vi "FFT on FPGA (BUGGED!).vi"   [LabVIEW 2014]
uses:
  <vilib>/Platform/TimedLoop/XDataNode/timing_clust.ctl
  <vilib>/Platform/TimedLoop/XDataNode/nitl_modes.ctl
  <vilib>/Platform/TimedLoop/XDataNode/wakeup.ctl
  <vilib>/rvi/Analysis/measure/FFT/simModelSupport/niFPGA FFT Streaming Sim Properties.ctl
  <vilib>/rvi/Analysis/measure/FFT/simModelSupport/niFPGA FFT Sim Stream Group Properties.ctl
  <vilib>/rvi/Analysis/measure/FFT/simModelSupport/niFPGA FFT Sim Types.ctl
  <vilib>/rvi/Analysis/measure/FFT/simModelSupport/niFpgaFFTSimArithmeticProperties.ctl
  <vilib>/rvi/Analysis/measure/FFT/simModelSupport/niFpgaFFTSimDfxp.ctl
  <vilib>/fxp/LVFixedPointQuantizationPolicyTypeDef.ctl
  <vilib>/rvi/Analysis/measure/FFT/XNode/niFpgaFFTButterflyDelays.ctl
  <vilib>/rvi/Emulation/niFpgaSctlEmulationGetInTimedLoop.vi
  <vilib>/rvi/Emulation/niFpgaEmulationReportErrorSimple.vi
  <vilib>/rvi/Emulation/niFpgaGetClockAttributes.vi
  <vilib>/rvi/Emulation/niFpgaCriticalErrorInLSC.vi
  <vilib>/rvi/Emulation/niFpgaEmulationIsFPGAContextNoSignature.vi
  <vilib>/rvi/errors/niFpgaSetErrorForExecOnDevCompSimple.vi
  <vilib>/rvi/eio/common/nirviEmuReportErrorAndStop.vi
  <vilib>/rvi/DataTransferAndStorage/Container/Common/niFpgaContainerGetUniqueNameForEmu.vi
  <vilib>/rvi/FIFO/Fifo_Resource/nirvififoEmulationSetSize.vi
  <vilib>/rvi/FIFO/Fifo_Resource/nirviFifoEmulationQueueMgr.vi
  <instcachedir>/0/nirviFifoEmulationQueueMgr_E5CAEC123FF24DC58D834DCA3CDAA9B5.lvgen/nirviFifoEmulationQueueMgr_E5CAEC123FF24DC58D834DCA3CDAA9B5_012.vi
  <vilib>/rvi/FIFO/Fifo_Resource/nirvififoEmulationCreateLock.vi
  <vilib>/rvi/Emulation/niFpgaProcessEmulError.vi
  <vilib>/rvi/FIFO/Fifo_Resource/nirvififoEmulationObtainLock.vi
  <vilib>/rvi/FIFO/Fifo_Resource/nirvififoEmulationReleaseLock.vi
  <vilib>/rvi/occurrence/nirviWaitOnOccurrenceBase.vi
  <vilib>/rvi/errors/nirviReportUnexpectedCaseInternalError.vi
  <vilib>/rvi/errors/nirviReportUnexpectedCaseInternalError (U32).vi
  <vilib>/rvi/Memory/Memory_Emulation/niFpgaMemoryEmulationCacheClearOnFirstRun.vi
  <vilib>/rvi/Memory/Memory_Emulation/nirvimemoryEmulationManagerCache_MakeExclusive.vi
  <vilib>/rvi/Memory/Memory_Emulation/niFpgaMemoryEmulationValidateCache.vi
  <vilib>/rvi/Memory/Memory_Emulation/nirvimemoryEmulationManagerCache_InsertValue.vi
  <vilib>/Utility/error.llb/Clear Errors.vi
  <vilib>/rvi/Memory/Memory_Emulation/nirvimemoryEmulationManagerCache_ReleaseExclusive.vi
  <vilib>/rvi/Memory/Memory_Emulation/nirvimemoryEmulationManagerCache_GetValue.vi
  <vilib>/rvi/Memory/Memory_Emulation/nirvimemoryEmulationManagerCache_SetValue.vi
  <instcachedir>/0/nirviFifoEmulationQueueMgr_E5CAEC123FF24DC58D834DCA3CDAA9B5.lvgen/nirviFifoEmulationQueueMgr_E5CAEC123FF24DC58D834DCA3CDAA9B5_010.vi
  <vilib>/rvi/eio/common/nirviEmuTemplateMethod_errors.vi
  <vilib>/rvi/FIFO/Fifo_Resource/nirvififoEmulationDetermineInputValidOut.vi
  <vilib>/rvi/Memory/Memory_Emulation/nirvimemoryFastEmulation.vi
  <vilib>/rvi/Memory/Memory_Emulation/nirvimemoryEmulation.vi
  <vilib>/rvi/interface/RandomDataEmulation/niFpgaRandomDataHandleErrors.vi
  <vilib>/rvi/Analysis/measure/FFT/simModelSupport/niFpgaFFTSimModelStreamingCore.vi
  <vilib>/Platform/TimedLoop/XDataNode/XDataNode.xnode
  <vilib>/rvi/DataTransferAndStorage/Container/XNode/niFpgaContainer.xnode
  <vilib>/rvi/FIFO/Fifo_Resource/nirvififoEmulationRead.vi
  <vilib>/rvi/DataTransferAndStorage/Register/Emulation/niFpgaRegisterEmulation.vi
  <vilib>/eio/EIOMethodNode/EIOMethodNode.xnode
  <vilib>/rvi/FIFO/Fifo_Resource/nirvififoEmulationWrite.vi
  <vilib>/rvi/interface/RandomDataEmulation/nirviRandomDataFpgaReadWriteTemplate.vi
  <vilib>/rvi/Analysis/measure/FFT/XNode/niFpgaFFT.xnode
  <vilib>/Platform/TimedLoop/XDataNode/XDNodeRunTimeDep.lvlib
types:
  T1 = typedef "XDNodeRunTimeDep.lvlib/timing_clust.ctl" = cluster{"Expected End [f-1]":u64, "Actual End [f-1]":u64, "Finished Late? [f-1]":bool, "Expected End [i-1]":u64, "Actual End [i-1]":u64, "Finished Late? [i-1]":bool, "Expected Start [i]":u64, "Actual Start [i]":u64, "Expected Start [f]":u64, "Actual Start [f]":u64, "Source Name":string, "Structure Name":string, "Period":i64, "Deadline":i64, "Offset":i64, "Start":i64, "Priority":i32, "Timeout":i32, "Mode":T2, "Wakeup Reason":T3, "Error":errorcluster, "Source Type":string, "Secondary Source Type":string, "Global End Time":u64, "Global Start Time":u64, "Frame Duration":u64, "Iteration Duration":u64, "Assigned CPU":i32, "I/O Scan Engine Mode":u32}
  T2 = typedef "XDNodeRunTimeDep.lvlib/nitl_modes.ctl" = enum32{"No Change", "Process missed periods, maintain original phase", "Discard missed periods, maintain original phase", "Process missed periods, ignore original phase", "Discard missed periods, ignore original phase"}
  T3 = typedef "XDNodeRunTimeDep.lvlib/wakeup.ctl" = enum32{"Normal", "Aborted", "Asynchronous wakeup", "Timing source error", "Timed loop error", "Timeout"}
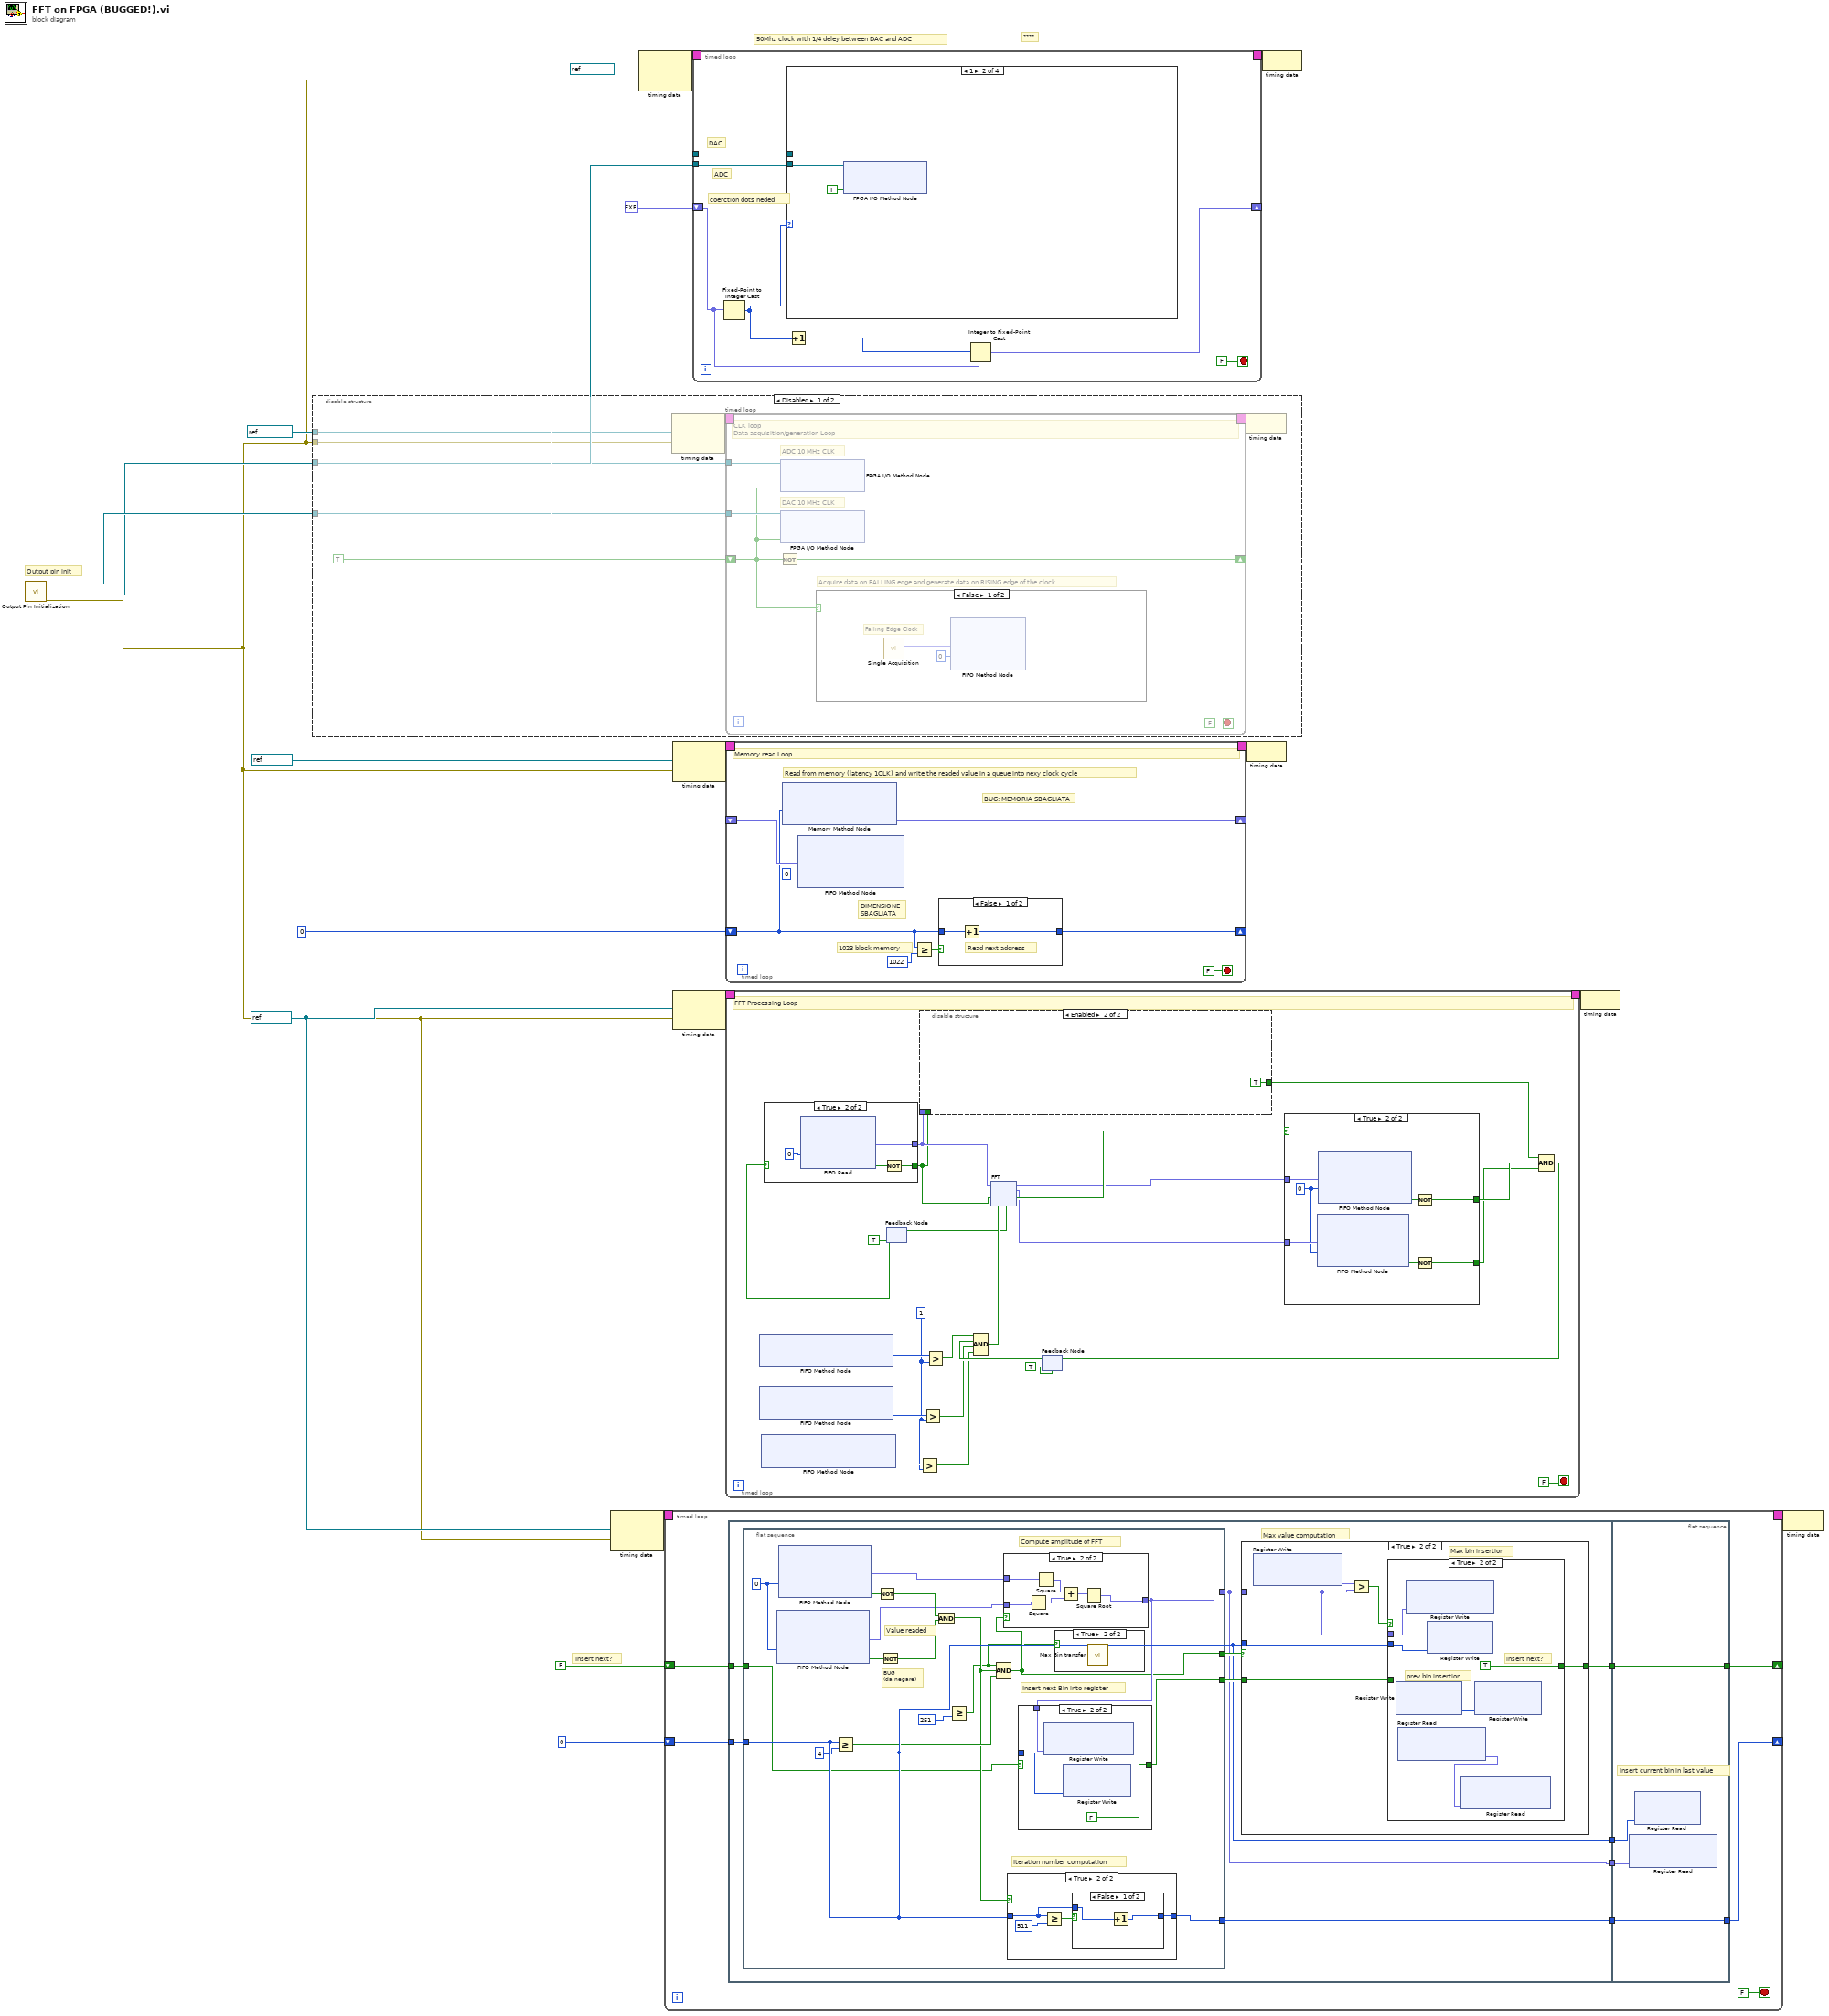
[diagram p0: block diagram]
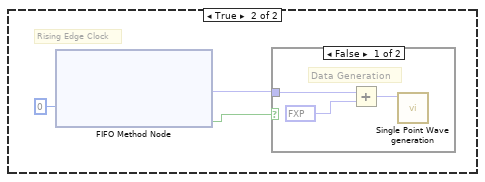
[diagram p2: hidden frame]
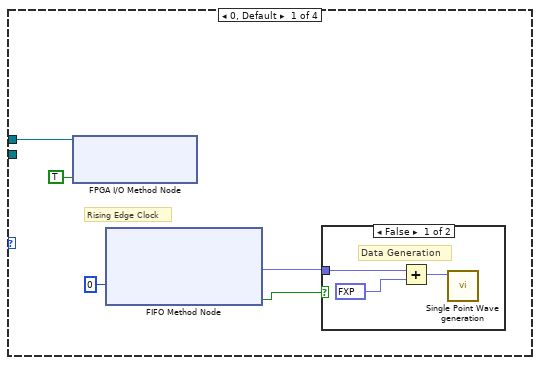
[diagram p5: hidden frame]
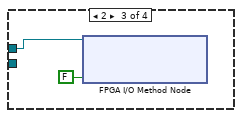
[diagram p7: hidden frame]
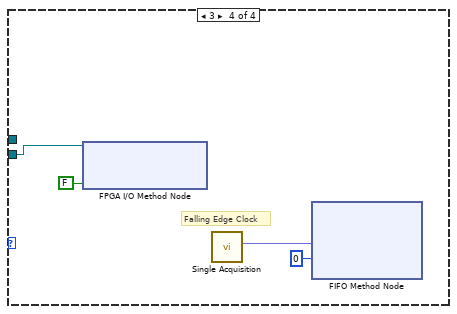
[diagram p8: hidden frame]
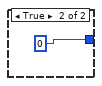
[diagram p12: hidden frame]
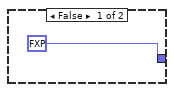
[diagram p13: hidden frame]
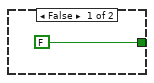
[diagram p15: hidden frame]
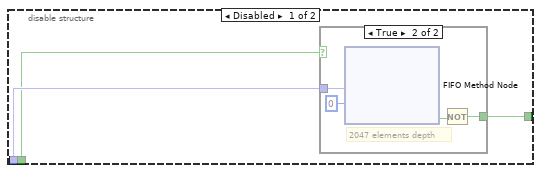
[diagram p16: hidden frame]
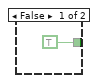
[diagram p17: hidden frame]
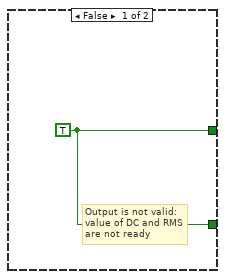
[diagram p18: hidden frame]
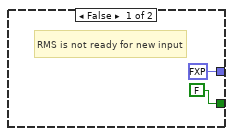
[diagram p19: hidden frame]
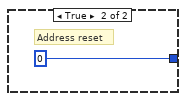
[diagram p20: hidden frame]
diagram:
  w10 = refnum<k21> "50MHz" ("Source Name")
  # "????"
  # "50Mhz clock with 1/4 deley between DAC and ADC"
  # "Insert next?"
  # "Output pin init"
  n1 = call "Output Pin Initialization.vi"() -> ("error out"=w1:errorcluster, "I/O Out Clock DAC (pin16)"=w2:refnum<k21>, "I/O Out Clock ADC (pin17)"=w3:refnum<k21>)  [unwired: 8 in]
  n2 = disable-structure shown="Disabled" {
    disable-tunnel: w1 -> [w23 _]
    disable-tunnel: refnum<k21> "100MHz" ("Source Name") -> [w22 _]
    disable-tunnel: w3 -> [w21 _]
    disable-tunnel: w2 -> [w20 _]
    frame Disabled {
      n3 = node-c288(w22, w23) -> (w26:T1)
      n4 = timed-loop {
        timing: w26 -> [_]
        timing-out: [_] -> w25
        shift-right: [w29] -> _
        shift-left: TRUE -> [w27]
        tunnel: w20 -> [w31]
        tunnel: w21 -> [w28]
        stop <- FALSE stop-if-true
        # "DAC 10 MHz CLK"
        # "Acquire data on FALLING edge and generate data on RISING edge of the clock"
        # "ADC 10 MHz CLK"
        # "CLK loop\nData acquisition/generation Loop"
        n5 = Not(x=w27) -> (.not. x?=w29:bool)
        n6 = xnode "FPGA I/O Method Node"("FPGA I/O In"=w31, "Data"=w27) -> ()  [unwired: 1 out]
        n7 = xnode "FPGA I/O Method Node"("FPGA I/O In"=w28, "Data"=w27) -> ()  [unwired: 1 out]
        n8 = case shown="False" w27 {
          frame False {
            # "Falling Edge Clock"
            n9 = call "Single Acquisition.vi"() -> ("Out"=w32:fxp<+/-,12,12>)  [unwired: 10 in, 1 out]
            n10 = xnode ("FIFO Method Node")("Element"=w32, "Timeout"=0) -> ()  [unwired: 1 in, 2 out]
          }
          frame True {
            # "Rising Edge Clock"
            n11 = xnode ("FIFO Method Node")("Timeout"=0) -> ("Element"=w34:fxp<+/-,12,12>, "Timed Out?"=w35:bool)  [unwired: 1 in, 1 out]
            n12 = case shown="False" w35 {
              tunnel: w34 -> [w39 _]
              frame False {
                # "Data Generation"
                n13 = Add(x=w39, y=fxp<+,12,12> 2048.0) -> (x+y=w37:fxp<+/-,14,14>)
                n14 = call "Single Point Wave generation.vi"("Data To Write"=w37) -> ()  [unwired: 10 in, 1 out]
              }
              frame True {
                # "FPGA memory slow"
              }
            }
          }
        }
      }
      n15 = node-c288(w25) -> ()
    }
    frame Enabled {
    }
  }
  n16 = node-c288(w10, w1) -> (w13:T1)
  n17 = node-c288(refnum<k21> "200MHz" ("Source Name"), w1) -> (w8:T1)
  n18 = timed-loop {
    timing: w13 -> [_]
    timing-out: [_] -> w12
    shift-right: [w54] -> _
    shift-left: 0 ("Timeout") -> [w51]
    shift-right: [w53] -> _
    shift-left: FALSE -> [w52]
    stop <- FALSE stop-if-true
    n19 = flat-sequence {
      tunnel: [w61] -> w49
      tunnel: [w60] -> w48
      tunnel: [w56] -> w47
      tunnel: [w57] -> w50
      tunnel: w52 -> [w59]
      tunnel: w51 -> [w57]
      tunnel: [w115] -> w53
      tunnel: [w116] -> w54
      tunnel: w49 -> [w116]
      tunnel: w48 -> [w115]
      tunnel: w47 -> [w114]
      tunnel: w50 -> [w113]
      frame #0 {
        # "Max value computation"
        n20 = flat-sequence {
          tunnel: [w65] -> w62
          tunnel: [w71] -> w61
          tunnel: w59 -> [w63]
          tunnel: [w68] -> w58
          tunnel: [w67] -> w56
          tunnel: w57 -> [w66]
          frame #0 {
            w80 = 0 ("Timeout")
            # "BUG\n(da negare)"
            # "Iteration number computation"
            # "Insert next Bin into register"
            # "Compute amplitude of FFT"
            # "Value readed"
            n21 = xnode ("FIFO Method Node")("Timeout"=w80) -> ("Element"=w69:fxp<+/-,22,22>, "Timed Out?"=w78:bool)  [unwired: 1 in, 1 out]
            n22 = xnode ("FIFO Method Node")("Timeout"=w80) -> ("Element"=w75:fxp<+/-,22,22>, "Timed Out?"=w79:bool)  [unwired: 1 in, 1 out]
            n23 = Greater Or Equal?(x=w66, y=4) -> (x >= y?=w73:bool)
            n24 = Not(x=w79) -> (.not. x?=w77:bool)
            n25 = Not(x=w78) -> (.not. x?=w76:bool)
            n26 = And(x=w77, y=w76) -> (x .and. y?=w72:bool)
            n27 = Greater Or Equal?(x=w66, y=251) -> (x >= y?=w64:bool)
            n28 = Compound Arithmetic op=AND(w64, w72, w73) -> (w65:bool)
            n29 = case shown="True" w65 {
              tunnel: w75 -> [_ w99]
              tunnel: w69 -> [_ w98]
              tunnel: [fxp<+,46,22> 0.0 w94] -> w67
              frame False {
              }
              frame True {
                n30 = Square(x=w98) -> (x^2=w96:fxp<+,43,43>)
                n31 = Square(x=w99) -> (x^2=w97:fxp<+,43,43>)
                n32 = Add(x=w97, y=w96) -> (x+y=w95:fxp<+,44,44>)
                n33 = Square Root(x=w95) -> (sqrt(x)=w94:fxp<+,46,22>)
              }
            }
            n34 = case shown="True" w72 {
              tunnel: w66 -> [w85 w87]
              tunnel: [w85 w86] -> w71
              frame False {
              }
              frame True {
                n35 = Greater Or Equal?(x=w87, y=511) -> (x >= y?=w89:bool)
                n36 = case shown="False" w89 {
                  tunnel: w87 -> [w90 _]
                  tunnel: [w91 0 ("Timeout")] -> w86
                  frame False {
                    n37 = Increment(x=w90) -> (x+1=w91:i32)
                  }
                  frame True {
                  }
                }
              }
            }
            n38 = case shown="True" w63 {
              selector: w63 -> [w81 _]
              tunnel: [w81 FALSE] -> w68
              tunnel: w67 -> [_ w83]
              tunnel: w66 -> [_ w84]
              frame False {
              }
              frame True {
                n39 = xnode "Register Write"("Data"=w83) -> ()  [unwired: 1 in, 1 out]
                n40 = xnode "Register Write"("Data"=w84) -> ()  [unwired: 1 in, 1 out]
              }
            }
            n41 = case shown="True" w64 {
              frame False {
              }
              frame True {
                n42 = call "Max Bin transfer.vi"() -> ()  [unwired: 11 in, 1 out]
              }
            }
          }
        }
        n43 = case shown="True" w62 {
          tunnel: w56 -> [_ w104]
          tunnel: w57 -> [_ w103]
          tunnel: [w100 w102] -> w60
          tunnel: w58 -> [w100 w101]
          frame False {
          }
          frame True {
            # "Max bin insertion"
            n44 = xnode "Register Write"() -> ("Data"=w106:fxp<+,46,22>)  [unwired: 1 in, 1 out]
            n45 = Greater?(x=w106, y=w104) -> (0:w105:bool)
            n46 = case shown="True" w105 {
              tunnel: w104 -> [_ w112]
              tunnel: w103 -> [_ w111]
              tunnel: [FALSE TRUE] -> w102
              tunnel: w101 -> [_ _]
              frame False {
              }
              frame True {
                # "insert next?"
                # "prev bin insertion"
                n47 = xnode "Register Write"() -> ("Data"=w109:i32)  [unwired: 1 in, 1 out]
                n48 = xnode "Register Read"() -> ("Data"=w108:fxp<+,46,22>)  [unwired: 1 in, 1 out]
                n49 = xnode "Register Write"("Data"=w112) -> ()  [unwired: 1 in, 1 out]
                n50 = xnode "Register Write"("Data"=w111) -> ()  [unwired: 1 in, 1 out]
                n51 = xnode "Register Read"("Data"=w108) -> ()  [unwired: 1 in, 1 out]
                n52 = xnode "Register Write"("Data"=w109) -> ()  [unwired: 1 in, 1 out]
              }
            }
          }
        }
      }
      frame #1 {
        # "Insert current bin in last value"
        n53 = xnode "Register Read"("Data"=w114) -> ()  [unwired: 1 in, 1 out]
        n54 = xnode "Register Read"("Data"=w113) -> ()  [unwired: 1 in, 1 out]
      }
    }
  }
  n55 = node-c288(refnum<k21> "50MHz" ("Source Name"), w1) -> (w19:T1)
  n56 = node-c288(w10, w1) -> (w17:T1)
  n57 = timed-loop {
    timing: w8 -> [_]
    timing-out: [_] -> w7
    shift-right: [w119] -> _
    shift-left: fxp<+,2,2> 0.0 -> [w120]
    tunnel: w3 -> [w124]
    tunnel: w2 -> [w123]
    stop <- FALSE stop-if-true
    # "ADC"
    # "DAC"
    # "coerction dots neded"
    n58 = Fixed-Point to Integer Cast(1:w120) -> (0:w122:u8)
    n59 = case shown="1" w122 {
      tunnel: w124 -> [w130 _ w137 _]
      tunnel: w123 -> [_ w135 _ w141]
      frame 0, Default {
        # "Rising Edge Clock"
        n60 = xnode "FPGA I/O Method Node"("FPGA I/O In"=w130, "Data"=TRUE) -> ()  [unwired: 1 out]
        n61 = xnode ("FIFO Method Node")("Timeout"=0) -> ("Element"=w126:fxp<+/-,12,12>, "Timed Out?"=w127:bool)  [unwired: 1 in, 1 out]
        n62 = case shown="False" w127 {
          tunnel: w126 -> [w133 _]
          frame False {
            # "Data Generation"
            n63 = Add(x=w133, y=fxp<+,12,12> 2048.0) -> (x+y=w131:fxp<+/-,14,14>)
            n64 = call "Single Point Wave generation.vi"("Data To Write"=w131) -> ()  [unwired: 10 in, 1 out]
          }
          frame True {
            # "FPGA memory slow"
          }
        }
      }
      frame 1 {
        n65 = xnode "FPGA I/O Method Node"("FPGA I/O In"=w135, "Data"=TRUE) -> ()  [unwired: 1 out]
      }
      frame 2 {
        n66 = xnode "FPGA I/O Method Node"("FPGA I/O In"=w137, "Data"=FALSE) -> ()  [unwired: 1 out]
      }
      frame 3 {
        # "Falling Edge Clock"
        n67 = xnode "FPGA I/O Method Node"("FPGA I/O In"=w141, "Data"=FALSE) -> ()  [unwired: 1 out]
        n68 = call "Single Acquisition.vi"() -> ("Out"=w138:fxp<+/-,12,12>)  [unwired: 10 in, 1 out]
        n69 = xnode ("FIFO Method Node")("Element"=w138, "Timeout"=0) -> ()  [unwired: 1 in, 2 out]
      }
    }
    n70 = Increment(x=w122) -> (x+1=w121:u8)
    n71 = Integer to Fixed-Point Cast(fixed-point type=w120, integer=w121) -> (fixed-point=w119:fxp<+,2,2>)
  }
  n72 = timed-loop {
    timing: w19 -> [_]
    timing-out: [_] -> w18
    shift-right: [w151] -> _
    shift-left: _ -> [w147]
    shift-right: [w148] -> _
    shift-left: u32 0 -> [w144]
    stop <- FALSE stop-if-true
    # "DIMENSIONE \nSBAGLIATA"
    # "BUG: MEMORIA SBAGLIATA"
    # "1023 block memory"
    # "Read from memory (latency 1CLK) and write the readed value in a queue into nexy clock cycle"
    # "Memory read Loop"
    n73 = xnode ("Memory Method Node")("Address"=w144) -> ("Data"=w151:fxp<+/-,12,12>)  [unwired: 1 in, 1 out]
    n74 = xnode ("FIFO Method Node")("Element"=w147, "Timeout"=0) -> ()  [unwired: 1 in, 2 out]
    n75 = Greater Or Equal?(x=w144, y=u32 1022) -> (x >= y?=w149:bool)
    n76 = case shown="False" w149 {
      tunnel: w144 -> [w153 _]
      tunnel: [w152 u32 0] -> w148
      frame False {
        # "Read next address"
        n77 = Increment(x=w153) -> (x+1=w152:u32)
      }
      frame True {
        # "Address reset"
      }
    }
  }
  n78 = timed-loop {
    timing: w17 -> [_]
    timing-out: [_] -> w16
    stop <- FALSE stop-if-true
    w159 = u32 1 ("y")
    # "FFT Processing Loop"
    n79 = xnode ("FIFO Method Node")() -> ("Number of Elements to Write"=w176:u32)  [unwired: 1 in, 1 out]
    n80 = xnode ("FIFO Method Node")() -> ("Number of Elements to Write"=w161:u32)  [unwired: 1 in, 1 out]
    n81 = xnode ("FIFO Method Node")() -> ("Number of Elements to Write"=w160:u32)  [unwired: 1 in, 1 out]
    n82 = feedback #1(TRUE ("ready for input")) -> (w179:bool)
    n83 = case shown="True" w179 {
      tunnel: [FALSE w228] -> w171
      tunnel: [fxp<+/-,12,12> 0.0 ("Element") w225] -> w172
      frame False {
        # "RMS is not ready for new input"
      }
      frame True {
        n84 = xnode ("FIFO Read")("Timeout"=0) -> ("Element"=w225:fxp<+/-,12,12>, "Timed Out?"=w227:bool)  [unwired: 1 in, 1 out]
        n85 = Not(x=w227) -> (.not. x?=w228:bool)
      }
    }
    n86 = disable-structure shown="Enabled" {
      disable-tunnel: w172 -> [w182 _]
      disable-tunnel: w171 -> [w181 _]
      disable-tunnel: [w180 TRUE] -> w165
      frame Disabled {
        n87 = case shown="True" w181 {
          tunnel: w182 -> [_ w187]
          tunnel: [TRUE w184] -> w180
          frame False {
          }
          frame True {
            # "2047 elements depth"
            n88 = xnode ("FIFO Method Node")("Element"=w187, "Timeout"=0) -> ("Timed Out?"=w185:bool)  [unwired: 1 in, 1 out]
            n89 = Not(x=w185) -> (.not. x?=w184:bool)
          }
        }
      }
      frame Enabled {
      }
    }
    n90 = Greater?(x=w160, y=w159) -> (0:w157:bool)
    n91 = Greater?(x=w161, y=w159) -> (0:w158:bool)
    n92 = Greater?(x=w176, y=w159) -> (0:w175:bool)
    n93 = feedback #2(TRUE) -> (w173:bool)
    n94 = Compound Arithmetic op=AND(w175, w173, w158, w157) -> (w170:bool)
    n95 = xnode "FFT"("real data in"=w172, "input valid"=w171, "ready for output"=w170) -> ("ready for input"=w169:bool, "real data out"=w167:fxp<+/-,22,22>, "imaginary data out"=w166:fxp<+/-,22,22>, "output valid"=w168:bool)  [unwired: 2 in, 1 out]
    n96 = feedback-in #1(w169) -> ()
    n97 = case shown="True" w168 {
      tunnel: w167 -> [_ w222]
      tunnel: w166 -> [_ w221]
      tunnel: [w215 w220] -> w164
      tunnel: [w215 w219] -> w163
      frame False {
        w215 = TRUE
        # "Output is not valid:\nvalue of DC and RMS\nare not ready"
      }
      frame True {
        w216 = 0 ("Timeout")
        n98 = xnode ("FIFO Method Node")("Element"=w221, "Timeout"=w216) -> ("Timed Out?"=w218:bool)  [unwired: 1 in, 1 out]
        n99 = xnode ("FIFO Method Node")("Element"=w222, "Timeout"=w216) -> ("Timed Out?"=w217:bool)  [unwired: 1 in, 1 out]
        n100 = Not(x=w217) -> (.not. x?=w220:bool)
        n101 = Not(x=w218) -> (.not. x?=w219:bool)
      }
    }
    n102 = Compound Arithmetic op=AND(w165, w164, w163) -> (w162:bool)
    n103 = feedback-in #2(w162) -> ()
  }
  n104 = node-c288(w18) -> ()
  n105 = node-c288(w7) -> ()
  n106 = node-c288(w16) -> ()
  n107 = node-c288(w12) -> ()
